vi "BRig_dataLC_Wrong_nRew2_l2.vi"() -> (2 "output_Wrong_nRew2_l2":i32)   [LabVIEW 2014]
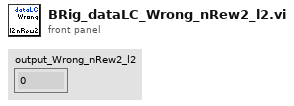
[diagram p1: front panel]
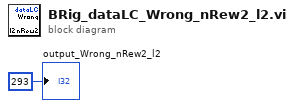
[diagram p0: block diagram]
diagram:
  "output_Wrong_nRew2_l2" <- 293 ("output_iBlock")
